vi "Main.vi"() -> ()   [LabVIEW 2012]
doc: "This sample project is built upon the standard state machine template and shows how you could create an application that acquires, analyzes, and presents data. It includes functionality for presenting configuration dialogs, preserving settings between executions, loading and saving data, as well as exporting graph images and text files.\n\nIt is most appropriate for data that is acquired instantly as it does not allow for screen updates mid acquisition nor does it allow for continuous streaming to disk."
uses:
  controls/State.ctl
  controls/Data.ctl
  controls/UI References.ctl
  controls/Graph Data.ctl
  <vilib>/Utility/miscctls.llb/LVAnnotationListTypeDef.ctl
  <vilib>/Utility/miscctls.llb/LVCursorListTypeDef.ctl
  controls/User Specified Data.ctl
  controls/HW Configuration.ctl
  controls/Simulated Signal Type.ctl
  controls/Analysis Configuration.ctl
  controls/New Data Behavior.ctl
panel:
  in  "Settings":bool
  in  "Snapshot":bool
  in  "Analyze":bool
  in  "Clear":bool
  in  "Stop":bool
  in  "Acquire":bool
  in  "Export":bool
  in  "Save Data":bool
  in  "Load Data":bool
  out "Boolean":bool
  out "Graph":waveform(dbl)[](graph)
  out "Status Bar":string
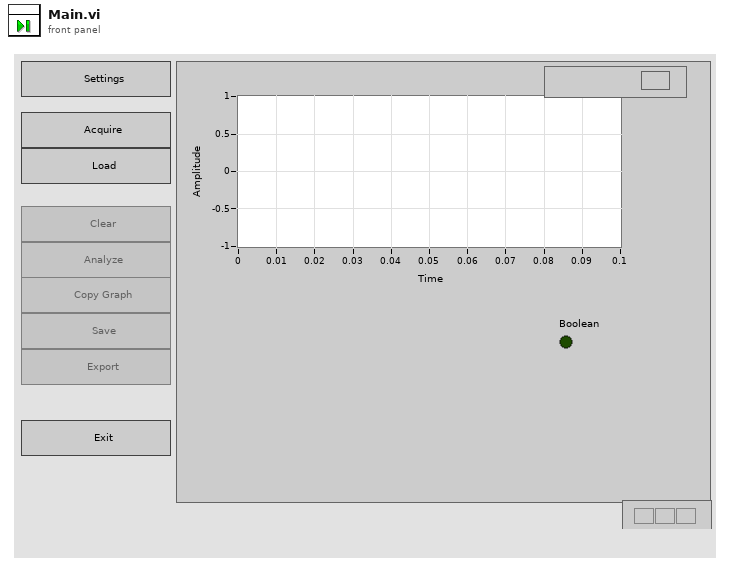
[diagram p1: front panel]
types:
  T1 = typedef "Data.ctl" = cluster{"UI References":T2, "Graph Data":T3, "User Specified":T6}
  T2 = typedef "UI References.ctl" = cluster{"Stop Ref":refnum<vi>, "Save Ref":refnum<vi>, "Open Ref":refnum<vi>, "Export Ref":refnum<vi>, "Acquire Ref":refnum<vi>, "Configure Ref":refnum<vi>, "Graph Ref":refnum<vi>, "Clear Ref":refnum<vi>, "Analyze Ref":refnum<vi>, "Status Ref":refnum<vi>, "Snapshot Ref":refnum<vi>}
  T3 = typedef "Graph Data.ctl" = cluster{"Data":waveform(dbl)[], "Annotation List":T4, "Cursor List":T5, "Analysis Data":waveform(dbl)[]}
  T4 = typedef "LVAnnotationListTypeDef.ctl" = cluster{"Name":string, "Color":u32, "Style":u8, "Point Style":u8, "Name Visible":bool, "Allow Drag":bool, "Annotation Mode":u32, "Plot":i32, "Index":i32, "Position":cluster{"X":dbl, "Y":dbl}, "X Scale":u32, "Y Scale":u32, "Show Arrow":bool, "Lock Name":bool, "Plot Area":i32, "Label Offset":cluster{"X":dbl, "Y":dbl}}[]
  T5 = typedef "LVCursorListTypeDef.ctl" = cluster{"Name":string, "Color":u32, "Style":u8, "Point Style":u8, "Name Visible":bool, "Allow Drag":bool, "Cursor Mode":u32, "Plot":i32, "Index":i32, "Position":cluster{"X":dbl, "Y":dbl}, "X Scale":u32, "Y Scale":u32, "Watch Plots":i32[], "Watch All Plots":bool, "Plot Area":i32, "Label Offset":cluster{"X":dbl, "Y":dbl}}[]
  T6 = typedef "User Specified Data.ctl" = cluster{"Hardware Configuration":T7, "Analysis Configuration":T9, "New Data Behavior":T10}
  T7 = typedef "HW Configuration.ctl" = cluster{"HW Refnum <Replace Me>":string, "Signal Type <Replace Me>":T8}
  T8 = typedef "Simulated Signal Type.ctl" = enum16{"Sine Wave", "Square Wave"}
  T9 = typedef "Analysis Configuration.ctl" = cluster{"Statistics":bool}
  T10 = typedef "New Data Behavior.ctl" = enum16{"Replace", "Overlay", "Append"}
  T11 = typedef "State.ctl" = enum16{"Initialize", "Wait for Event", "Update UI", "Configure", "Acquire", "Load Data", "Save Data", "Clear Data", "Export Data", "Analyze", "Copy Graph", "Stop"}
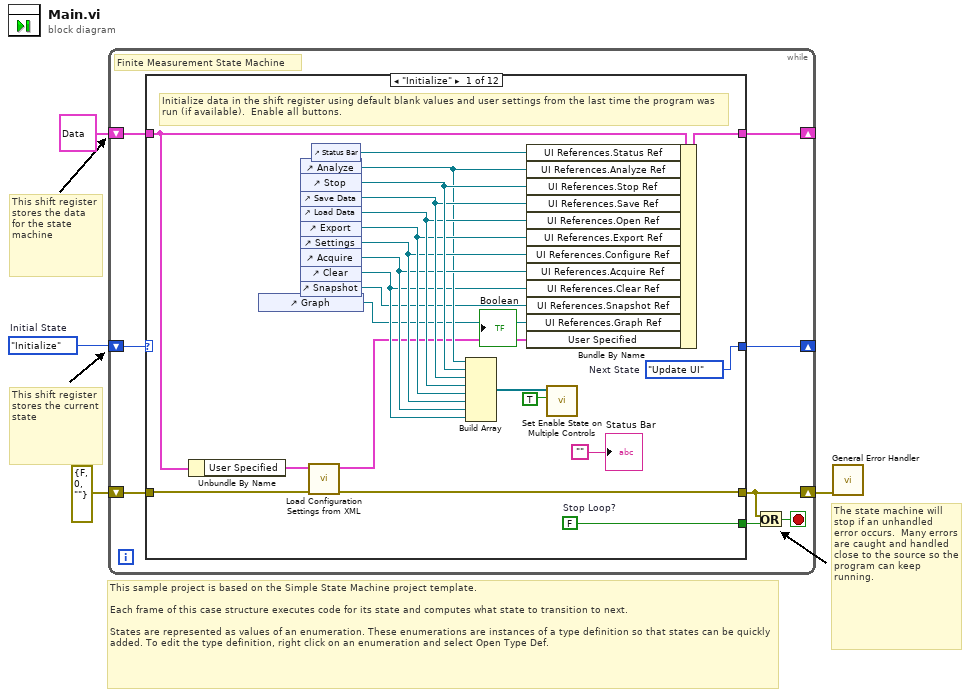
[diagram p0: block diagram]
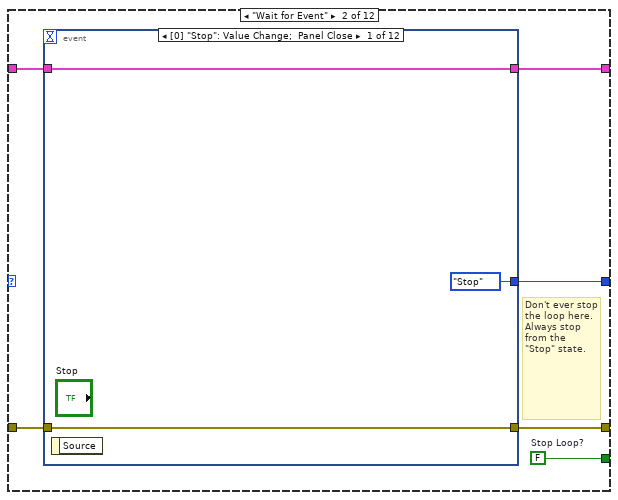
[diagram p2: hidden frame]
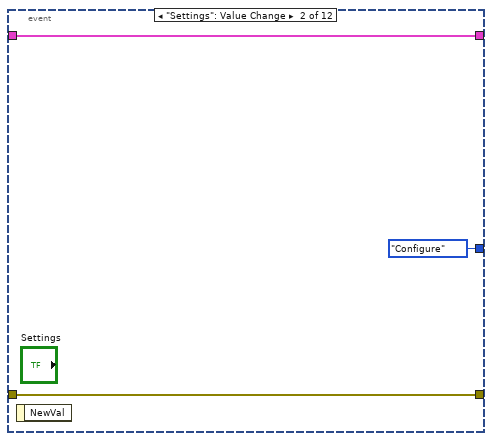
[diagram p3: hidden frame]
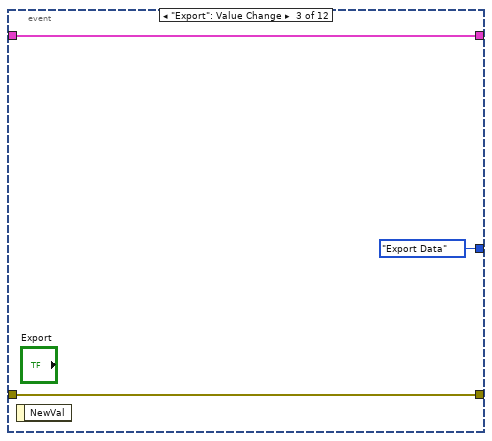
[diagram p4: hidden frame]
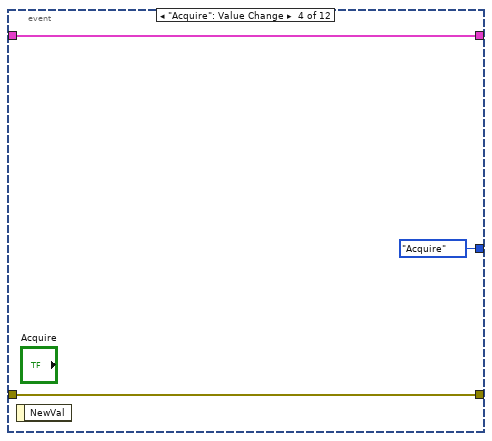
[diagram p5: hidden frame]
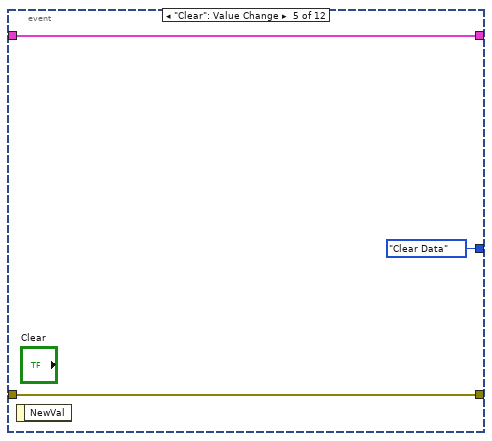
[diagram p6: hidden frame]
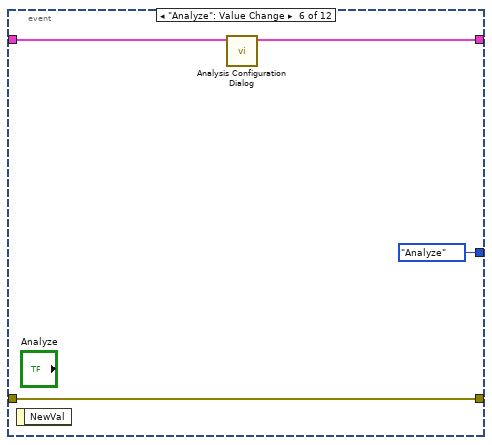
[diagram p7: hidden frame]
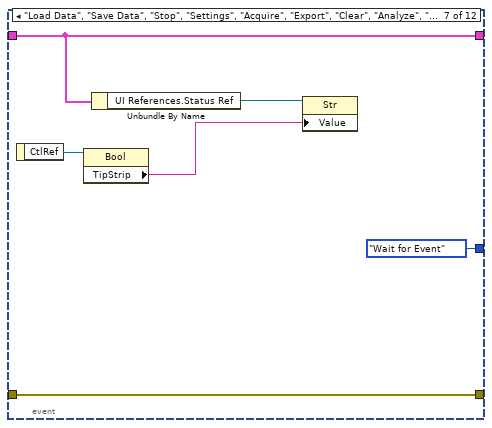
[diagram p8: hidden frame]
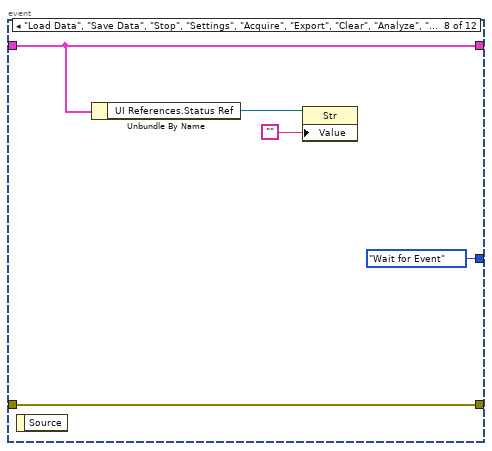
[diagram p9: hidden frame]
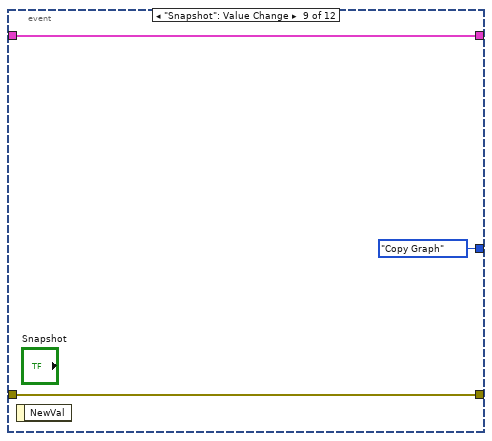
[diagram p10: hidden frame]
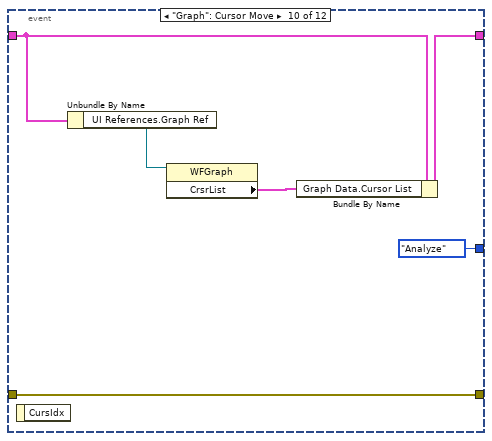
[diagram p11: hidden frame]
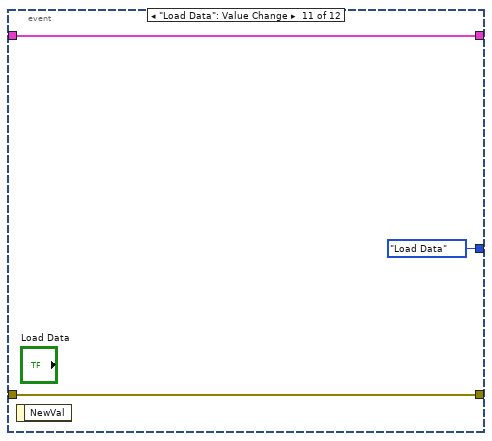
[diagram p12: hidden frame]
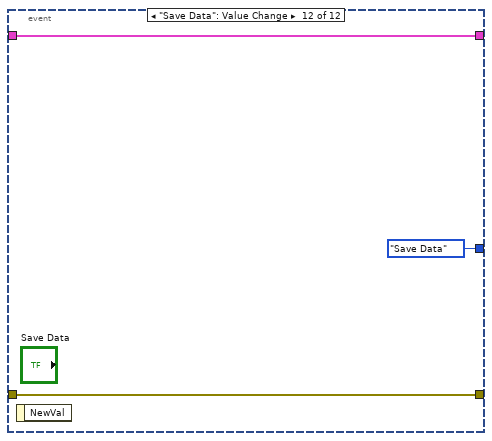
[diagram p13: hidden frame]
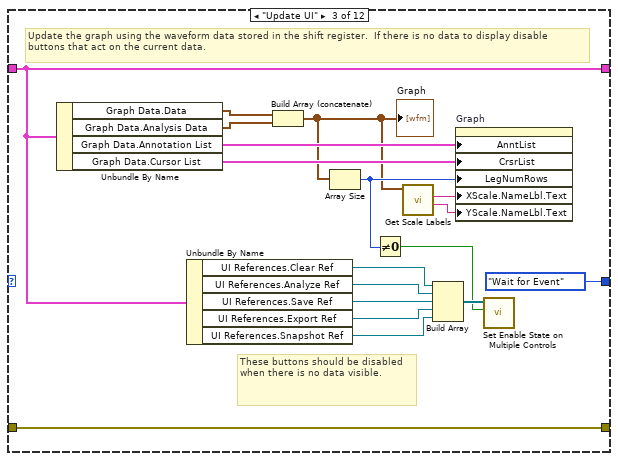
[diagram p14: hidden frame]
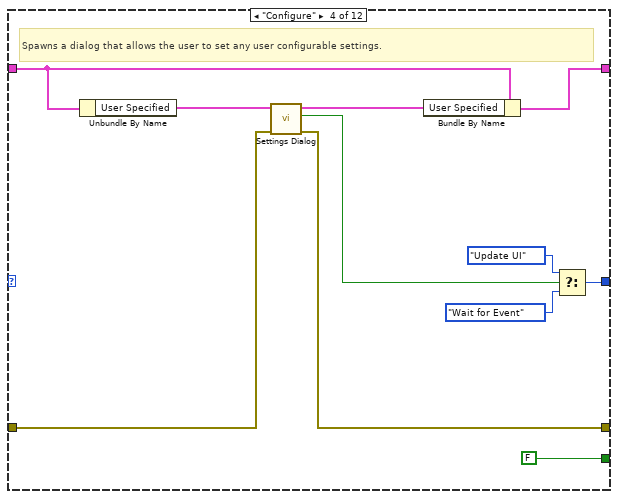
[diagram p15: hidden frame]
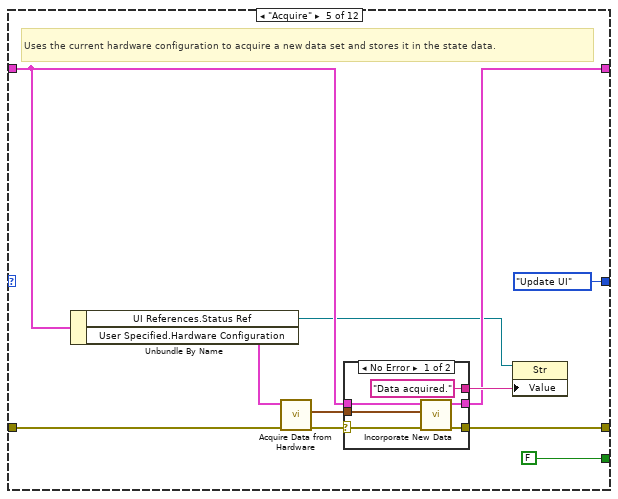
[diagram p16: hidden frame]
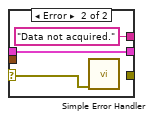
[diagram p17: hidden frame]
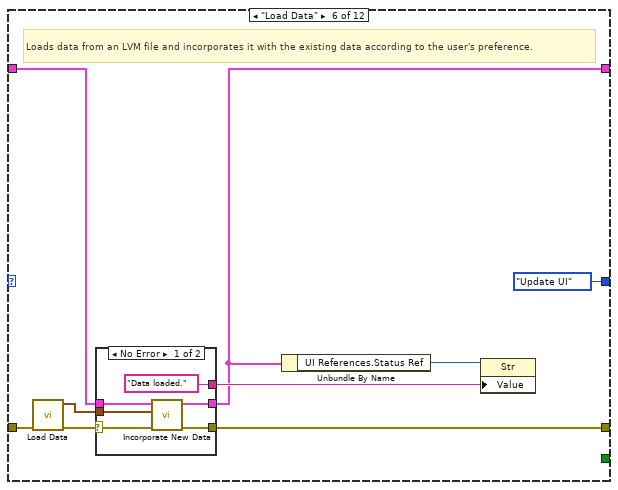
[diagram p18: hidden frame]
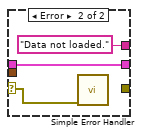
[diagram p19: hidden frame]
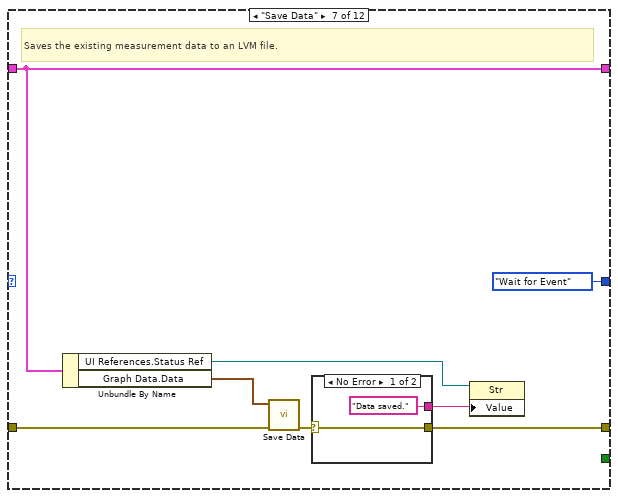
[diagram p20: hidden frame]
diagram:
  w4 = State."Initialize"  # Initial State
  # "The state machine will stop if an unhandled error occurs.  Many errors are caught and handled close to the source so the program can keep running."
  # "This shift register\nstores the data for the state machine"
  # "This sample project is based on the Simple State Machine project template.\n\nEach frame of this case structure executes code for its state and computes what state to transition to next.\n\nStates are represented as values of an enumeration. These enumerations are instances of a type definition so that states can be quickly added. To edit the type definition, right click on an enumeration and select Open Type Def."
  # "This shift register\nstores the current\nstate"
  n1 = while {
    shift-right: [w11] -> _
    shift-left: w4 -> [w12]
    shift-right: [w9] -> _
    shift-left: T1 {"UI References"={"Stop Ref"=refnum, "Save Ref"=refnum, "Open Ref"=refnum, "Export Ref"=refnum, "Acquire Ref"=refnum, "Configure Ref"=refnum, "Graph Ref"=refnum, "Clear Ref"=refnum, "Analyze Ref"=refnum, "Status Ref"=refnum, "Snapshot Ref"=refnum}, "Graph Data"={"Data"=[], "Annotation List"=[], "Cursor List"=[], "Analysis Data"=[]}, "User Specified"={"Hardware Configuration"={"HW Refnum <Replace Me>"="", "Signal Type <Replace Me>"=enum."Sine Wave"}, "Analysis Configuration"={"Statistics"=FALSE}, "New Data Behavior"=enum."Replace"}} ("Data") -> [w10]
    shift-right: [w5] -> w1
    shift-left: errorcluster {"status"=FALSE, "code"=0, "source"=""} ("error constant") -> [w8]
    stop <- w6 stop-if-true
    # "Finite Measurement State Machine"
    n2 = case shown="\"Initialize\"" w12 {
      tunnel: [w34 w40 State."Wait for Event" ("(Value Not Used)") w107 State."Update UI" ("Next State") State."Update UI" ("(Value Not Used)") State."Wait for Event" ("(Value Not Used)") State."Wait for Event" ("(Value Not Used)") State."Update UI" ("(Value Not Used)") State."Update UI" ("(Value Not Used)") State."Wait for Event" ("(Value Not Used)") w197] -> w11
      tunnel: [w33 w39 _ FALSE ("Stop Loop?") FALSE ("Stop Loop?") _ _ _ _ _ _ w196] -> w7
      tunnel: w10 -> [w24 w38 w100 w113 w120 w143 w156 w168 w179 w182 w188 w194]
      tunnel: [w32 w37 w100 w112 w119 w137 w156 w168 w178 w182 w188 w194] -> w9
      tunnel: w8 -> [w22 w36 w103 w111 w122 w142 w158 w171 w181 w183 w187 w191]
      tunnel: [w21 w35 w103 w110 w115 w141 w154 w165 w181 w183 w186 w190] -> w5
      frame "Initialize" {
        w33 = FALSE  # Stop Loop?
        w34 = State."Update UI"  # Next State
        # "Initialize data in the shift register using default blank values and user settings from the last time the program was run (if available).  Enable all buttons."
        n3 = Unbundle By Name(w24) -> ("User Specified"=w23:T6)
        n4 = control-ref of="Graph"() -> (w13:refnum<vi>)
        n5 = control-ref of="Analyze"() -> (w20:refnum<vi>)
        n6 = control-ref of="Stop"() -> (w31:refnum<vi>)
        n7 = control-ref of="Save Data"() -> (w30:refnum<vi>)
        n8 = control-ref of="Load Data"() -> (w29:refnum<vi>)
        n9 = control-ref of="Export"() -> (w28:refnum<vi>)
        n10 = control-ref of="Settings"() -> (w27:refnum<vi>)
        n11 = control-ref of="Acquire"() -> (w26:refnum<vi>)
        n12 = control-ref of="Clear"() -> (w18:refnum<vi>)
        n13 = control-ref of="Snapshot"() -> (w14:refnum<vi>)
        n14 = call "Load Configuration Settings from XML.vi"("error in (no error)"=w22, "User Configuration in"=w23) -> ("error out"=w21:errorcluster, "User Configuration out"=w16:T6)  [unwired: 8 in]
        n15 = control-ref of="Status Bar"() -> (w19:refnum<vi>)
        n16 = Build Array(w20, w31, w30, w29, w28, w27, w26, w18) -> (w25:refnum<vi>[])
        n17 = Bundle By Name(cluster=w24, "UI References.Status Ref"=w19, "UI References.Analyze Ref"=w20, "UI References.Stop Ref"=w31, "UI References.Save Ref"=w30, "UI References.Open Ref"=w29, "UI References.Export Ref"=w28, "UI References.Configure Ref"=w27, "UI References.Acquire Ref"=w26, "UI References.Clear Ref"=w18, "UI References.Snapshot Ref"=w14, "UI References.Graph Ref"=w13, "User Specified"=w16) -> (w32:T1)
        n18 = call "Set Enable State on Multiple Controls.vi"("Enable?"=TRUE, "Controls"=w25) -> ()  [unwired: 10 in]
        "Status Bar" <- "" ("Status Bar")
      }
      frame "Wait for Event" {
        w39 = FALSE  # Stop Loop?
        # "Don't ever stop the loop here. Always stop from the \"Stop\" state."
        n19 = event shown="[0] \"Stop\": Value Change;  Panel Close" {
          selector: _ -> [_ _ _ _ _ _ _ _ _ _ _ _]
          dyn-events: _ -> [_ _ _ _ _ _ _ _ _ _ _ _]
          timeout: _ -> [_ _ _ _ _ _ _ _ _ _ _ _]
          tunnel: [State."Stop" ("Next State") State."Configure" ("Next State") State."Export Data" ("Next State") State."Acquire" ("Next State") State."Clear Data" ("Next State") State."Analyze" ("Next State") State."Wait for Event" ("Next State") State."Wait for Event" ("Next State") State."Copy Graph" ("Next State") State."Analyze" ("Next State") State."Load Data" ("Next State") State."Save Data" ("Next State")] -> w40
          tunnel: w38 -> [w42 w46 w49 w52 w55 w57 w63 w69 w73 w74 w81 w84]
          tunnel: [w42 w46 w49 w52 w55 w56 w63 w69 w73 w77 w81 w84] -> w37
          tunnel: w36 -> [w41 w45 w48 w51 w54 w59 w65 w70 w72 w79 w80 w83]
          tunnel: [w41 w45 w48 w51 w54 w59 w65 w70 w72 w79 w80 w83] -> w35
          event "Stop": Value Change; Panel Close {
            n20 = event-data() -> ()  [unwired: 1 in, 1 out]
          }
          event "Settings": Value Change {
            n21 = event-data() -> ()  [unwired: 1 in, 1 out]
          }
          event "Export": Value Change {
            n22 = event-data() -> ()  [unwired: 1 in, 1 out]
          }
          event "Acquire": Value Change {
            n23 = event-data() -> ()  [unwired: 1 in, 1 out]
          }
          event "Clear": Value Change {
            n24 = event-data() -> ()  [unwired: 1 in, 1 out]
          }
          event "Analyze": Value Change {
            n25 = event-data() -> ()  [unwired: 1 in, 1 out]
            n26 = call "Analysis Configuration Dialog.vi"("Data in"=w57) -> ("Data out"=w56:T1)  [unwired: 10 in]
          }
          event "Load Data", "Save Data", "Stop", "Settings", "Acquire", "Export", "Clear", "Analyze", "Snapshot": Mouse Enter {
            n27 = event-data() -> ("CtlRef"=w64:refnum<vi>)  [unwired: 1 in]
            n28 = property class="Bool"(reference=w64) -> ("TipStrip"=w61:string)  [unwired: 1 in, 2 out]
            n29 = Unbundle By Name(w63) -> ("UI References.Status Ref"=w62:refnum<vi>)
            n30 = property class="Str"(reference=w62, "Value"=w61) -> ()  [unwired: 1 in, 2 out]
          }
          event "Load Data", "Save Data", "Stop", "Settings", "Acquire", "Export", "Clear", "Analyze", "Snapshot": Mouse Leave {
            n31 = event-data() -> ()  [unwired: 1 in, 1 out]
            n32 = Unbundle By Name(w69) -> ("UI References.Status Ref"=w68:refnum<vi>)
            n33 = property class="Str"(reference=w68, "Value"="") -> ()  [unwired: 1 in, 2 out]
          }
          event "Snapshot": Value Change {
            n34 = event-data() -> ()  [unwired: 1 in, 1 out]
          }
          event "Graph": Cursor Move {
            n35 = event-data() -> ()  [unwired: 1 in, 1 out]
            n36 = Unbundle By Name(w74) -> ("UI References.Graph Ref"=w76:refnum<vi>)
            n37 = property class="WFGraph"(reference=w76) -> ("CrsrList"=w75:T5)  [unwired: 1 in, 2 out]
            n38 = Bundle By Name(cluster=w74, "Graph Data.Cursor List"=w75) -> (w77:T1)
          }
          event "Load Data": Value Change {
            n39 = event-data() -> ()  [unwired: 1 in, 1 out]
          }
          event "Save Data": Value Change {
            n40 = event-data() -> ()  [unwired: 1 in, 1 out]
          }
        }
      }
      frame "Update UI" {
        # "These buttons should be disabled when there is no data visible."
        # "Update the graph using the waveform data stored in the shift register.  If there is no data to display disable buttons that act on the current data."
        n41 = Unbundle By Name(w100) -> ("Graph Data.Data"=w96:waveform(dbl)[], "Graph Data.Analysis Data"=w86:waveform(dbl)[], "Graph Data.Annotation List"=w101:T4, "Graph Data.Cursor List"=w97:T5)
        n42 = Unbundle By Name(w100) -> ("UI References.Clear Ref"=w92:refnum<vi>, "UI References.Analyze Ref"=w91:refnum<vi>, "UI References.Save Ref"=w99:refnum<vi>, "UI References.Export Ref"=w89:refnum<vi>, "UI References.Snapshot Ref"=w90:refnum<vi>)
        n43 = Build Array (concatenate)(w96, w86) -> (w94:waveform(dbl)[])
        "Graph" <- w94
        n44 = Array Size(array=w94) -> (size(s)=w95:i32)
        n45 = Not Equal To 0?(x=w95) -> (x != 0?=w93:bool)
        n46 = call "Get Scale Labels.vi"("Array of Waveforms"=w94) -> ("Y Scale Label Text"=w87:string, "X Scale Label Text"=w88:string)  [unwired: 9 in]
        n47 = Build Array(w92, w91, w99, w89, w90) -> (w98:refnum<vi>[])
        n48 = property on="Graph" class="WFGraph (strict)"("AnntList"=w101, "CrsrList"=w97, "LegNumRows"=w95, "XScale.NameLbl.Text"=w88, "YScale.NameLbl.Text"=w87) -> ()  [unwired: 2 in, 2 out]
        n49 = call "Set Enable State on Multiple Controls.vi"("Enable?"=w93, "Controls"=w98) -> ()  [unwired: 10 in]
      }
      frame "Configure" {
        # "Spawns a dialog that allows the user to set any user configurable settings."
        n50 = Unbundle By Name(w113) -> ("User Specified"=w105:T6)
        n51 = call "Settings Dialog.vi"("error in (no error)"=w111, "Configuration in"=w105) -> ("error out"=w110:errorcluster, "UI Refresh Needed?"=w109:bool, "Configuration out"=w104:T6)  [unwired: 7 in]
        n52 = Bundle By Name(cluster=w113, "User Specified"=w104) -> (w112:T1)
        n53 = Select(t=State."Update UI" ("Next State if true"), s=w109, f=State."Wait for Event" ("Next State if false")) -> (s? t:f=w107:T11)
      }
      frame "Acquire" {
        # "Uses the current hardware configuration to acquire a new data set and stores it in the state data."
        n54 = Unbundle By Name(w120) -> ("UI References.Status Ref"=w116:refnum<vi>, "User Specified.Hardware Configuration"=w123:T7)
        n55 = call "Acquire Data from Hardware.vi"("error in (no error)"=w122, "Hardware Configuration"=w123) -> ("error out"=w117:errorcluster, "Graph Data"=w118:waveform(dbl)[])  [unwired: 7 in]
        n56 = case shown="No Error" w117 {
          selector: w117 -> [w128 w133]
          tunnel: w120 -> [w127 w134]
          tunnel: [w131 w134] -> w119
          tunnel: [w130 _] -> w115
          tunnel: w118 -> [w129 _]
          tunnel: ["Data acquired." ("Data acquired") "Data not acquired." ("Data not acquired")] -> w121
          frame No Error {
            n57 = call "Incorporate New Data.vi"("error in (no error)"=w128, "New Graph Data"=w129, "Data in"=w127) -> ("error out"=w130:errorcluster, "Data out"=w131:T1)  [unwired: 7 in]
          }
          frame Error {
            n58 = call <vilib>:"Simple Error Handler.vi"("error in (no error)"=w133) -> ()  [unwired: 4 in, 5 out]
          }
        }
        n59 = property class="Str"(reference=w116, "Value"=w121) -> ()  [unwired: 1 in, 2 out]
      }
      frame "Load Data" {
        # "Loads data from an LVM file and incorporates it with the existing data according to the user's preference."
        n60 = call "Load Data.vi"("error in (no error)"=w142) -> ("error out"=w139:errorcluster, "New Graph Data"=w136:waveform(dbl)[])  [unwired: 9 in]
        n61 = case shown="No Error" w139 {
          selector: w139 -> [w146 w151]
          tunnel: w143 -> [w145 w152]
          tunnel: [w149 w152] -> w137
          tunnel: [w148 _] -> w141
          tunnel: w136 -> [w147 _]
          tunnel: ["Data loaded." ("Data loaded") "Data not loaded." ("Data not loaded")] -> w138
          frame No Error {
            n62 = call "Incorporate New Data.vi"("error in (no error)"=w146, "New Graph Data"=w147, "Data in"=w145) -> ("error out"=w148:errorcluster, "Data out"=w149:T1)  [unwired: 7 in]
          }
          frame Error {
            n63 = call <vilib>:"Simple Error Handler.vi"("error in (no error)"=w151) -> ()  [unwired: 4 in, 5 out]
          }
        }
        n64 = Unbundle By Name(w137) -> ("UI References.Status Ref"=w135:refnum<vi>)
        n65 = property class="Str"(reference=w135, "Value"=w138) -> ()  [unwired: 1 in, 2 out]
      }
      frame "Save Data" {
        # "Saves the existing measurement data to an LVM file."
        n66 = Unbundle By Name(w156) -> ("UI References.Status Ref"=w155:refnum<vi>, "Graph Data.Data"=w159:waveform(dbl)[])
        n67 = call "Save Data.vi"("error in (no error)"=w158, "Data"=w159) -> ("error out"=w157:errorcluster)  [unwired: 9 in]
        n68 = case shown="No Error" w157 {
          selector: w157 -> [w161 w164]
          tunnel: ["Data saved." ("Data saved") "Data not saved." ("Data not saved")] -> w153
          tunnel: [w161 _] -> w154
          frame No Error {
          }
          frame Error {
            n69 = call <vilib>:"Simple Error Handler.vi"("error in (no error)"=w164) -> ()  [unwired: 4 in, 5 out]
          }
        }
        n70 = property class="Str"(reference=w155, "Value"=w153) -> ()  [unwired: 1 in, 2 out]
      }
      frame "Export Data" {
        # "Exports the currently loaded measurement and analysis data to a text file that can be imported into a spreadsheet or other application."
        n71 = Unbundle By Name(w168) -> ("UI References.Status Ref"=w166:refnum<vi>, "Graph Data"=w167:T3)
        n72 = call "Export Data.vi"("error in (no error)"=w171, "Graph Data"=w167) -> ("error out"=w169:errorcluster)  [unwired: 9 in]
        n73 = case shown="No Error" w169 {
          selector: w169 -> [w173 w176]
          tunnel: ["Data exported." ("Data exported") "Data not exported." ("Data not exported")] -> w170
          tunnel: [w173 _] -> w165
          frame No Error {
          }
          frame Error {
            n74 = call <vilib>:"Simple Error Handler.vi"("error in (no error)"=w176) -> ()  [unwired: 4 in, 5 out]
          }
        }
        n75 = property class="Str"(reference=w166, "Value"=w170) -> ()  [unwired: 1 in, 2 out]
      }
      frame "Clear Data" {
        # "Clears the data currently in the graph."
        n76 = Bundle By Name(cluster=w179, "Graph Data"=T3 {"Data"=[], "Annotation List"=[], "Cursor List"=[], "Analysis Data"=[]} ("Graph")) -> (w178:T1)
      }
      frame "Analyze" {
        # "Code Recommended - Add your own signal analysis here."
        # "Analyzes the measurement data."
        n77 = Unbundle By Name(w182) -> ("Graph Data"=w184:T3)
        n78 = call "Statistical Analysis.vi"("Graph Data In"=w184) -> ()  [unwired: 8 in, 2 out]
      }
      frame "Copy Graph" {
        # "Places an image of the graph on the clipboard for pasting into reports or emails."
        n79 = call "Copy Graph to Clipboard.vi"("error in (no error)"=w187, "Graph Data"=w188) -> ("error out"=w186:errorcluster)  [unwired: 9 in]
      }
      frame "Stop" {
        w196 = TRUE  # Stop Loop?
        w197 = State."Stop"  # (Value Not Used)
        # "Saves the users settings to an XML file and stops execution."
        # "The state value is not used here since this is the last iteration of the state machine loop"
        n80 = Unbundle By Name(w194) -> ("UI References.Status Ref"=w192:refnum<vi>, "User Specified"=w195:T6)
        n81 = call "Save Configuration Settings to XML.vi"("error in (no error)"=w191, "User Configuration"=w195) -> ("error out"=w190:errorcluster)  [unwired: 9 in]
        n82 = property class="Str"(reference=w192, "Value"="Stopped." ("Stopped")) -> ()  [unwired: 1 in, 2 out]
      }
    }
    n83 = Or(x=w5, y=w7) -> (x .or. y?=w6:bool)
  }
  n84 = call <vilib>:"General Error Handler.vi"("error in (no error)"=w1) -> ()  [unwired: 10 in, 5 out]
